vi "mod_QAM Transmitter.vi"(0 "Symbol Rate, Hz":dbl=1.0 format="%.2f", 1 "Reset?":bool=TRUE, 2 "# Samples per Symbol":i32=16, 5 "M-QAM":i32=16, 7 "Message":T2={"# Guard Bits"=4, "# Sync Bits"=40, "# Message Bits"=1000, "PN sequence order"=9}, 9 "System Filter":T1={"TX Filter"=enum."Root Raised Cos", "Alpha"=0.5, "filter length"=8} {"Alpha" format="%.2f"}, 11 "error in (no error)":errorcluster) -> (4 "Output Complex Waveform":T5 {"Y" format="%.3f"; "dt" format="%^.2e"; "t0" format="%.4f"}, 6 "Signal Description":T4 {"QAM System Parameters"."symbol map" format="%.3f"; "matched filter coefficients" format="%.2f"; "pulse shaping filter coefficients" format="%.2f"; "Sync (Symbols)" format="%.2f"}, 15 "error out":errorcluster)   [LabVIEW 2020, in "niDMT.lvlib"]
doc: "This example demonstrates generation of a QAM modulated signal. You can specify characteristics of the message signal such as PN sequence order, number of guard bits, number of sync bits, and transmit filter parameters. You can extend this example to download the generated QAM signal to GPIB-based RF signal generators."
uses:
  <vilib>/addons/Modulation/niDMT.lvlib
  <vilib>/addons/Modulation/Digital/Support/Controls/QAM System Parameters.ctl
  <vilib>/addons/Modulation/Analog/controls/Complex Data Waveform.ctl
  <vilib>/addons/Modulation/Analog/support/mod_Set Error Source.vi
  <vilib>/addons/Modulation/Digital/Support/Common/Validators/mod_Generate Filter Coefficients Validate.vi
  <vilib>/addons/Modulation/Digital/General/subVIs/mod_Generate Filter Coefficients.vi
  <vilib>/addons/Modulation/Digital/General/MT Generate QAM System Parameters(M).vi
  <vilib>/addons/Modulation/niAMT.lvlib
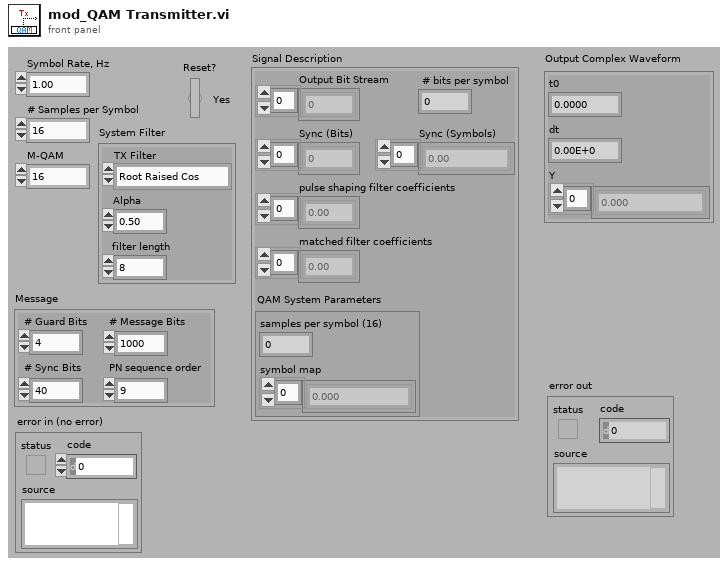
[diagram p1: front panel]
types:
  T1 = cluster{"TX Filter":enum16{"none", "Raised Cosine", "Root Raised Cos", "Gaussian"}, "Alpha":dbl, "filter length":i32}
  T2 = cluster{"# Guard Bits":i32, "# Sync Bits":i32, "# Message Bits":i32, "PN sequence order":i32}
  T3 = typedef "niDMT.lvlib/QAM System Parameters.ctl" = cluster{"samples per symbol (16)":i32, "symbol map":cdb[]}
  T4 = cluster{"Output Bit Stream":i8[], " # bits per symbol":i32, "Sync (Bits)":i8[], "Sync (Symbols)":cdb[], "pulse shaping filter coefficients":dbl[], "matched filter coefficients":dbl[], "QAM System Parameters":T3}
  T5 = typedef "niAMT.lvlib/Complex Data Waveform.ctl" = cluster{"t0":dbl, "dt":dbl, "Y":cdb[]}
  T6 = cluster{"Output Bit Stream":i8[], "# bits per symbol":i32, "Sync (Bits)":i8[], "Sync (Symbols)":cdb[], "pulse shaping filter coefficients":dbl[], "matched filter coefficients":dbl[], "QAM System Parameters":T3}
  T7 = enum16{"none", "Raised Cosine", "Root Raised Cos", "Gaussian"}
  T8 = cluster{"samples per symbol (16)":i32, "symbol map":cdb[]}
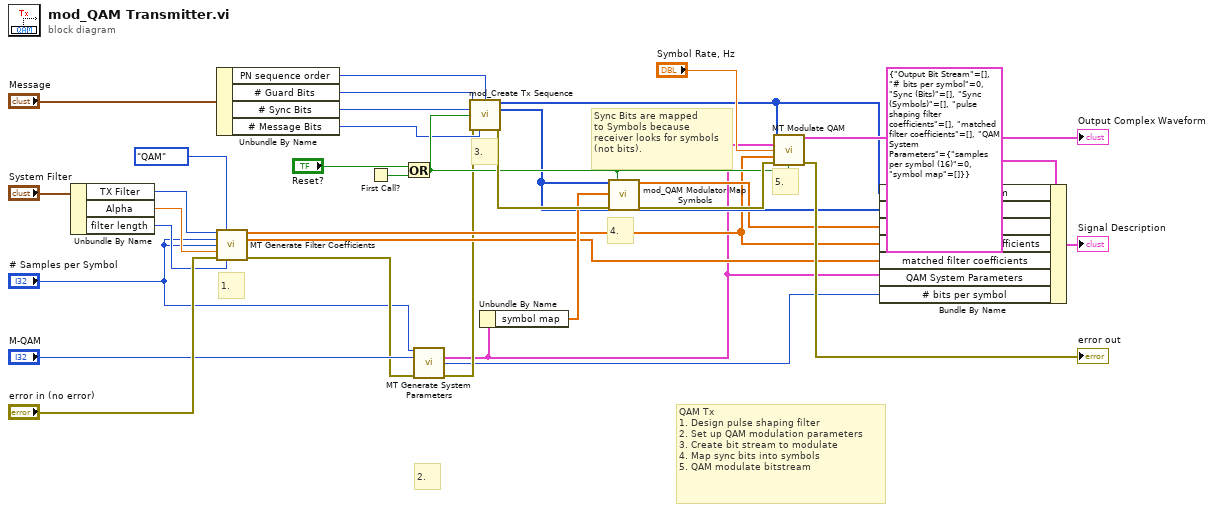
[diagram p0: block diagram]
diagram:
  # "5."
  # "4."
  # "2."
  # "3."
  # "1."
  # "QAM Tx\n1. Design pulse shaping filter\n2. Set up QAM modulation parameters\n3. Create bit stream to modulate\n4. Map sync bits into symbols\n5. QAM modulate bitstream"
  # "Sync Bits are mapped\nto Symbols because\nreceiver looks for symbols\n(not bits)."
  n1 = Unbundle By Name("System Filter") -> ("TX Filter"=w18:T7, "Alpha"=w17:dbl, "filter length"=w16:i32)
  n2 = Unbundle By Name("Message") -> ("PN sequence order"=w10:i32, "# Guard Bits"=w22:i32, "# Sync Bits"=w21:i32, "# Message Bits"=w20:i32)
  n3 = call <vilib>:"MT Generate Filter Coefficients.vi"("pulse shaping filter (none)"=w18, "modulation type"=enum16{"FSK", "PSK", "QAM", "MSK", "PAM", "ASK"}."QAM", "pulse shaping samples per symbol (16)"="# Samples per Symbol", "matched samples per symbol (16)"="# Samples per Symbol", "filter parameter"=w17, "error in (no error)"="error in (no error)", "filter length (symbols)"=w16) -> ("pulse shaping filter coefficients"=w12:dbl[], "matched filter coefficients"=w11:dbl[], "error out"=w6:errorcluster)  [unwired: 6 out]
  n4 = First Call?() -> (First Call?: T/F=w27:bool)
  n5 = Or(x="Reset?", y=w27) -> (x .or. y?=w25:bool)
  n6 = call-poly <vilib>:"MT Generate System Parameters.vi"("samples per symbol (16)"="# Samples per Symbol", "M-QAM (16)"="M-QAM", "error in (no error)"=w6) -> ("QAM system parameters"=w2:T8, "bits per symbol"=w3:i32, "error out"=w4:errorcluster)  [unwired: 10 out]
  n7 = call <vilib>:"mod_Create Tx Sequence.vi"("# Guard Bits (2)"=w22, "PN sequence order (9)"=w10, "# Sync Bits (20)"=w21, "Reset? (T)"=w25, "error in (no error)"=w4, "# Message Bits"=w20) -> ("Output Bit Stream"=w15:i8[], "Last Sync Pattern"=w14:i8[], "error out"=w31:errorcluster)  [unwired: 3 in, 4 out]
  n8 = Unbundle By Name(w2) -> ("symbol map"=w24:cdb[])
  n9 = call <vilib>:"mod_QAM Modulator Map Symbols.vi"("Input Bit Stream"=w14, "Symbol Map"=w24, "error in (no error)"=w31, "Reset? (T)"=w25) -> ("Symbols"=w13:cdb[], "error out"=w32:errorcluster)  [unwired: 10 out]
  n10 = call <vilib>:"MT Modulate QAM.vi"("input bit stream"=w15, "QAM system parameters"=w2, "symbol rate (Hz)"="Symbol Rate, Hz", "pulse shaping filter coefficients"=w12, "error in (no error)"=w32, "reset? (T)"=w25) -> ("output complex waveform"=→"Output Complex Waveform":T5, "error out"=→"error out":errorcluster)  [unwired: 1 in, 7 out]
  n11 = Bundle By Name(cluster=T6 {"Output Bit Stream"=[], "# bits per symbol"=0, "Sync (Bits)"=[], "Sync (Symbols)"=[], "pulse shaping filter coefficients"=[], "matched filter coefficients"=[], "QAM System Parameters"={"samples per symbol (16)"=0, "symbol map"=[]}} ("Signal Description"), "Output Bit Stream"=w15, "Sync (Bits)"=w14, "Sync (Symbols)"=w13, "pulse shaping filter coefficients"=w12, "matched filter coefficients"=w11, "QAM System Parameters"=w2, "# bits per symbol"=w3) -> (→"Signal Description":T6)
